vi "lfieldpanel_DO_disconnect.vi"(8 "error in (no error)":errorcluster, 11 "lightfield_panel in":refnum<class "lightfield_panel.lvclass">) -> (0 "error out":errorcluster, 3 "lightfield_panel out":refnum<class "lightfield_panel.lvclass">)   [LabVIEW 2015, in "lightfield_panel.lvclass"]
uses:
  lightfield_panel.lvclass
  lightfield/lightfield_class.lvclass
  UI/panel_class/panel.lvclass
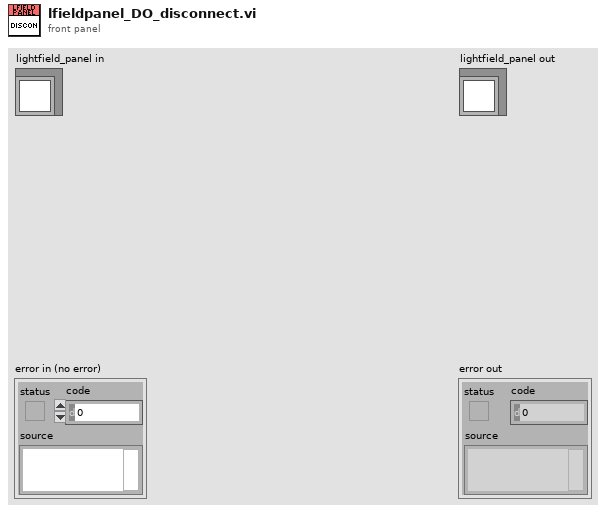
[diagram p1: front panel]
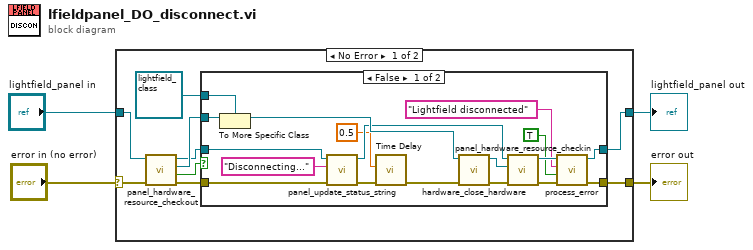
[diagram p0: block diagram]
diagram:
  n1 = case shown="No Error" "error in (no error)" {
    selector: "error in (no error)" -> [w12 w35]
    tunnel: [w6 w35] -> w3
    tunnel: [w5 w34] -> w1
    tunnel: "lightfield_panel in" -> [w13 w34]
    frame No Error {
      n2 = call "panel_hardware_resource_checkout.vi"("error in (no error)"=w12, "panel in"=w13) -> ("error out"=w8:errorcluster, "timed out?"=w11:bool, "hardware.lvclass"=w9:refnum<class "hardware.lvclass">, "panel out"=w7:refnum<class "lightfield_panel.lvclass">)  [unwired: 6 in]
      n3 = case shown="False" w11 {
        tunnel: refnum<class "lightfield_class.lvclass"> refnum ("lightfield_class.lvclass") -> [w31 _]
        tunnel: w9 -> [w30 _]
        tunnel: w8 -> [w20 w32]
        tunnel: w7 -> [w19 w33]
        tunnel: [w27 w32] -> w6
        tunnel: [w26 w33] -> w5
        frame False {
          n4 = To More Specific Class(target class=w31, reference=w30) -> (specific class reference=w23:refnum<class "lightfield_class.lvclass">)  [unwired: 1 in, 1 out]
          n5 = call-dynamic "panel_update_status_string.vi"("error in (no error)"=w20, "String"="Disconnecting...", "lightfield_panel in"=w19) -> ("error out"=w15:errorcluster, "lightfield_panel out"=w18:refnum<class "lightfield_panel.lvclass">)  [unwired: 7 in]
          n6 = call "Time Delay"("error in (no error)"=w15, "Delay Time (s)"=0.5) -> ("error out"=w14:errorcluster)  [unwired: 9 in]
          n7 = call-dynamic "hardware_close_hardware.vi"("error in (no error)"=w14, "lightfield_class in"=w23) -> ("error out"=w21:errorcluster, "lightfield_class out"=w22:refnum<class "lightfield_class.lvclass">)  [unwired: 8 in]
          n8 = call "panel_hardware_resource_checkin.vi"("error in (no error)"=w21, "hardware.lvclass"=w22, "panel in"=w18) -> ("error out"=w28:errorcluster, "panel out"=w29:refnum<class "lightfield_panel.lvclass">)  [unwired: 7 in]
          n9 = call "process_error.vi"("error in (no error)"=w28, "Update Status"=TRUE, "No Error Message"="Lightfield disconnected", "lightfield_panel in"=w29) -> ("error out"=w27:errorcluster, "lightfield_panel out"=w26:refnum<class "lightfield_panel.lvclass">)  [unwired: 6 in]
        }
        frame True {
        }
      }
    }
    frame Error {
    }
  }
  "error out" <- w3
  "lightfield_panel out" <- w1
